vi "NanonisFrame-Demod.vi"(0 "Positions":T1 {"z (mm)" format="%.1p"; "y (nm)" format="%.1p"; "x (nm)" format="%.1p"}, 2 "Signal":u16(ring) items=["Z Val", "Demod"]) -> (8 "X Out":dbl, 10 "Z Out":dbl, 11 "output cluster":T2, 12 "Speed":dbl, 14 "FO X":dbl, 15 "FO Z":dbl, 16 "FW":dbl, 17 "FH":dbl, 19 "CVAL (nA)":dbl)   [LabVIEW 2019]
uses:
  <userlib>/Nanonis Prog Interface V5/Nanonis Prog Interface.lvlib
panel:
  out "Signal value":sgl format="%#_6p"
  out "Signals Names":string[](array[string])
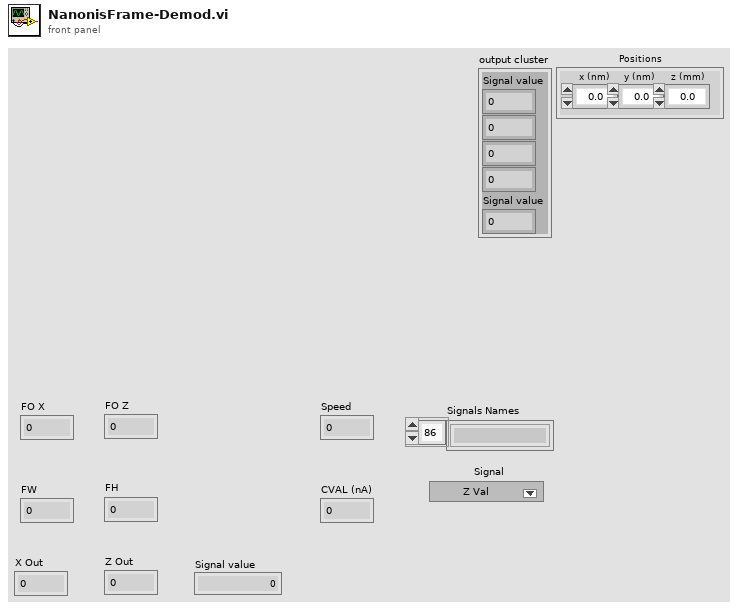
[diagram p1: front panel]
types:
  T1 = cluster{"x (nm)":dbl, "y (nm)":dbl, "z (mm)":dbl}
  T2 = cluster{"Signal value":sgl, dbl, dbl, dbl, "Signal value":sgl}
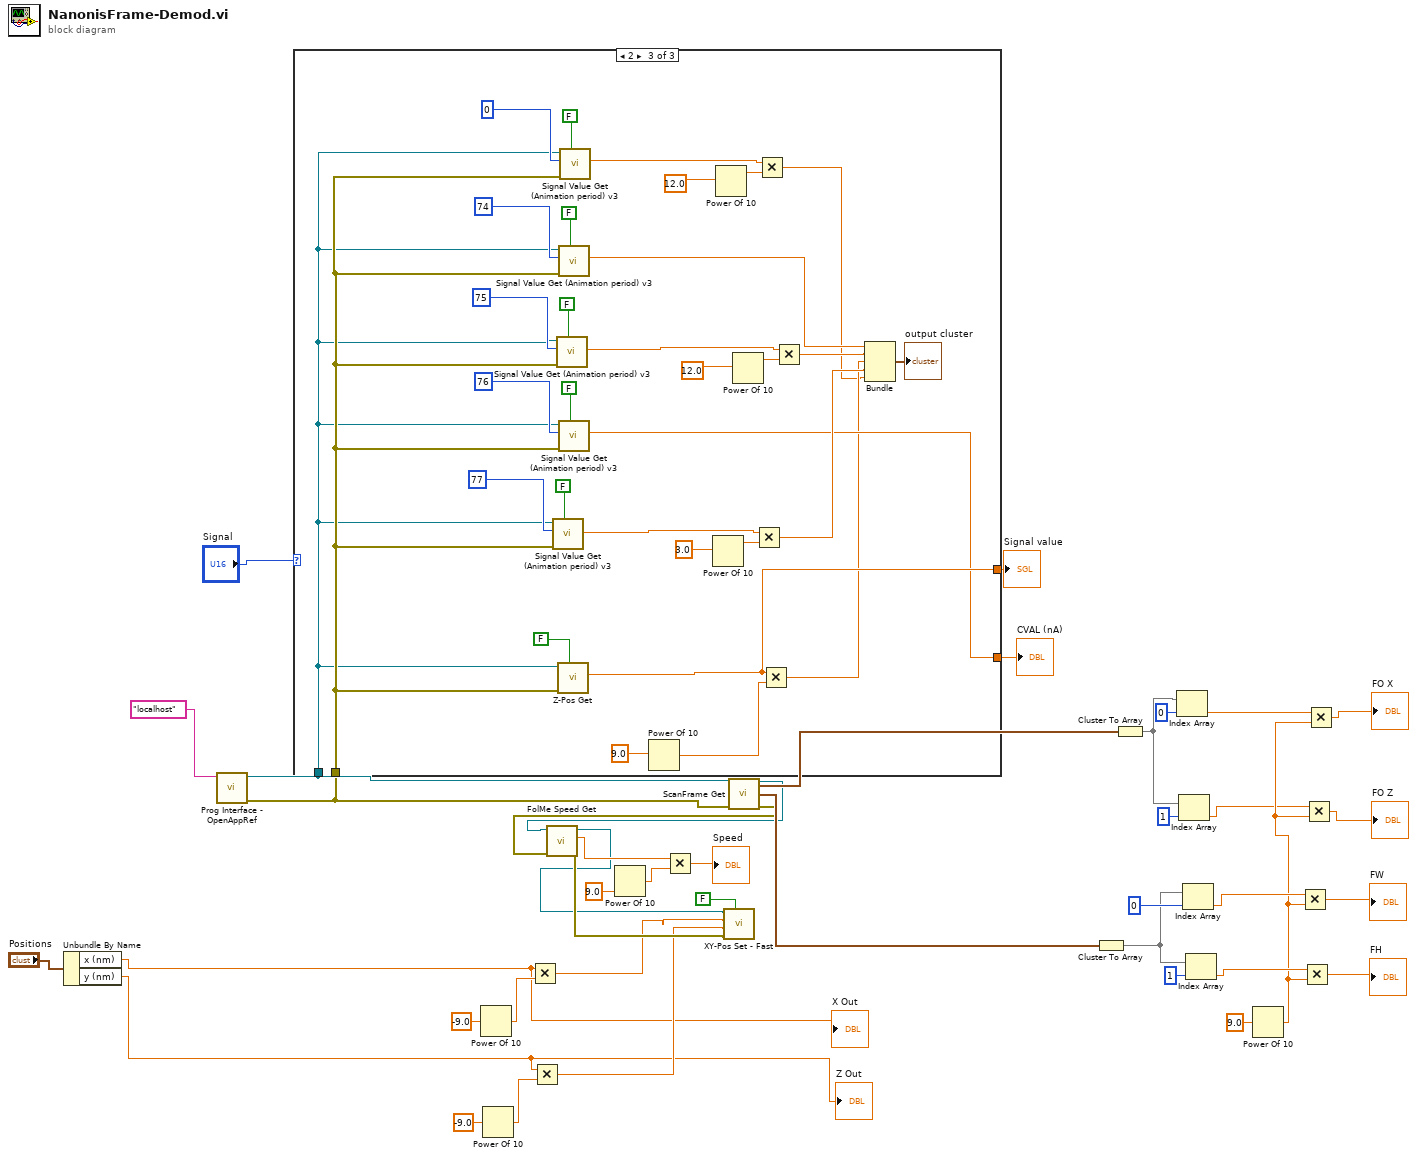
[diagram p0: block diagram]
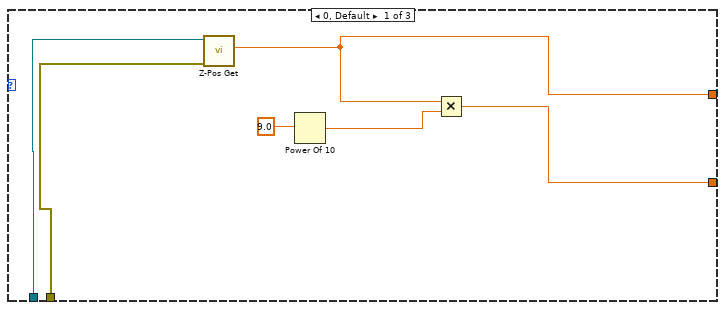
[diagram p2: hidden frame]
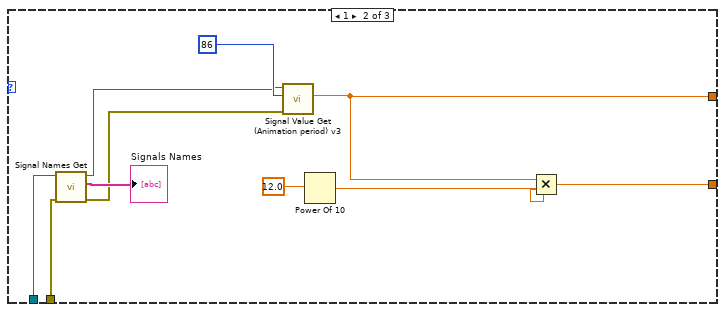
[diagram p3: hidden frame]
diagram:
  n1 = Unbundle By Name("Positions") -> ("x (nm)"=w2:dbl, "y (nm)"=w1:dbl)
  "X Out" <- w2
  "Z Out" <- w1
  n2 = call <userlib>:"Prog Interface - OpenAppRef.vi"("Machine name (local machine IP)"="localhost") -> ("Error out"=w6:errorcluster, "Application reference"=w7:refnum<vi>)  [unwired: 5 in]
  n3 = case shown="2" "Signal" {
    tunnel: [w46 w56 w69] -> w13
    tunnel: w7 -> [w44 w54 w64]
    tunnel: w6 -> [w43 w53 w65]
    tunnel: [w45 w49 w74] -> w5
    frame 0, Default {
      n4 = call <userlib>:"Z-Pos Get.vi"("error in (no error)"=w43, "Application ref in"=w44) -> ("Z position (m)"=w45:sgl)  [unwired: 7 in, 2 out]
      n5 = Power Of 10(x=9.0) -> (10^x=w48:dbl)
      n6 = Multiply(x=w45, y=w48) -> (x*y=w46:dbl)
    }
    frame 1 {
      n7 = call <userlib>:"Signal Names Get.vi"("error in (no error)"=w53, "Application ref in"=w54) -> ("error out"=w51:errorcluster, "Signals Names"=→"Signals Names":string[], "Application ref out"=w50:refnum<vi>)  [unwired: 5 in]
      n8 = call <userlib>:"Signal Value Get (Animation period) v3.vi"("error in (no error)"=w51, "Signal index (0-127)"=i8 86, "Application ref in"=w50) -> ("Signal value"=w49:sgl)  [unwired: 5 in, 2 out]
      n9 = Power Of 10(x=12.0) -> (10^x=w57:dbl)
      n10 = Multiply(x=w49, y=w57) -> (x*y=w56:dbl)
    }
    frame 2 {
      n11 = call <userlib>:"Signal Value Get (Animation period) v3.vi"("Wait for newest data (F=False)"=FALSE, "error in (no error)"=w65, "Signal index (0-127)"=i8 77, "Application ref in"=w64) -> ("Signal value"=w77:sgl)  [unwired: 4 in, 2 out]
      n12 = call <userlib>:"Signal Value Get (Animation period) v3.vi"("Wait for newest data (F=False)"=FALSE, "error in (no error)"=w65, "Signal index (0-127)"=i8 75, "Application ref in"=w64) -> ("Signal value"=w78:sgl)  [unwired: 4 in, 2 out]
      n13 = call <userlib>:"Z-Pos Get.vi"("Wait for newest data (F=False)"=FALSE, "error in (no error)"=w65, "Application ref in"=w64) -> ("Z position (m)"=w74:sgl)  [unwired: 6 in, 2 out]
      n14 = call <userlib>:"Signal Value Get (Animation period) v3.vi"("Wait for newest data (F=False)"=FALSE, "error in (no error)"=w65, "Signal index (0-127)"=i8 74, "Application ref in"=w64) -> ("Signal value"=w72:sgl)  [unwired: 4 in, 2 out]
      n15 = call <userlib>:"Signal Value Get (Animation period) v3.vi"("Wait for newest data (F=False)"=FALSE, "error in (no error)"=w65, "Signal index (0-127)"=i8 76, "Application ref in"=w64) -> ("Signal value"=w69:sgl)  [unwired: 4 in, 2 out]
      n16 = call <userlib>:"Signal Value Get (Animation period) v3.vi"("Wait for newest data (F=False)"=FALSE, "error in (no error)"=w65, "Signal index (0-127)"=i8 0, "Application ref in"=w64) -> ("Signal value"=w60:sgl)  [unwired: 4 in, 2 out]
      n17 = Power Of 10(x=9.0) -> (10^x=w76:dbl)
      n18 = Power Of 10(x=3.0) -> (10^x=w87:dbl)
      n19 = Power Of 10(x=12.0) -> (10^x=w61:dbl)
      n20 = Power Of 10(x=12.0) -> (10^x=w81:dbl)
      n21 = Multiply(x=w77, y=w87) -> (x*y=w70:dbl)
      n22 = Multiply(x=w60, y=w61) -> (x*y=w59:dbl)
      n23 = Multiply(x=w74, y=w76) -> (x*y=w68:dbl)
      n24 = Multiply(x=w78, y=w81) -> (x*y=w71:dbl)
      n25 = Bundle("Signal value"=w72, w71, w68, w70, w59) -> (→"output cluster":cluster{"Signal value":sgl, dbl, dbl, dbl, dbl})  [unwired: 1 in]
    }
  }
  "CVAL (nA)" <- w13
  "Signal value" <- w5
  n26 = Power Of 10(x=-9.0) -> (10^x=w22:dbl)
  n27 = Power Of 10(x=-9.0) -> (10^x=w20:dbl)
  n28 = Multiply(x=w2, y=w22) -> (x*y=w10:dbl)
  n29 = Multiply(x=w1, y=w20) -> (x*y=w11:dbl)
  n30 = Power Of 10(x=9.0) -> (10^x=w25:dbl)
  n31 = call <userlib>:"ScanFrame Get.vi"("Application ref in"=w7, "error in (no error)"=w6) -> ("Application ref out"=w27:refnum<vi>, "Center coordinates (m)"=w41:cluster{"Xc":sgl, "Yc":sgl}, "Size (m)"=w37:cluster{"Width":sgl, "Height":sgl}, "error out"=w18:errorcluster)  [unwired: 9 in, 1 out]
  n32 = call <userlib>:"FolMe Speed Get.vi"("error in (no error)"=w18, "Application ref in"=w27) -> ("error out"=w12:errorcluster, "Speed (m/s)"=w24:sgl, "Application ref out"=w9:refnum<vi>)  [unwired: 4 in, 1 out]
  n33 = Multiply(x=w24, y=w25) -> (x*y=→"Speed":dbl)
  n34 = call <userlib>:"XY-Pos Set - Fast.vi"("Wait end-of-motion (T=True)"=FALSE, "error in (no error)"=w12, "Y (m)"=w11, "X (m)"=w10, "Application ref in"=w9) -> ()  [unwired: 4 in, 2 out]
  n35 = Cluster To Array(cluster=w37) -> (array=w34:sgl[])
  n36 = Cluster To Array(cluster=w41) -> (array=w40:sgl[])
  n37 = Index Array(array=w40, index=0) -> (element=w15:sgl)
  n38 = Index Array(array=w40, index=1) -> (element=w14:sgl)
  n39 = Index Array(array=w34, index=0) -> (element=w33:sgl)
  n40 = Index Array(array=w34, index=1) -> (element=w32:sgl)
  n41 = Power Of 10(x=9.0) -> (10^x=w30:dbl)
  n42 = Multiply(x=w33, y=w30) -> (x*y=→"FW":dbl)
  n43 = Multiply(x=w32, y=w30) -> (x*y=→"FH":dbl)
  n44 = Multiply(x=w14, y=w30) -> (x*y=→"FO Z":dbl)
  n45 = Multiply(x=w15, y=w30) -> (x*y=→"FO X":dbl)
